vi "r3_HDI&sensor_position_theta.vi"() -> ()   [LabVIEW 2016]
uses:
  Classes/Controllers/Motion/Copy of Motion Folder/Motion.lvclass
  Classes/Controllers/Camera/Copy of Controller Folder/Controller.lvclass
panel:
  in  "Default sensor size type B size":dbl[](array[numeric])=[22.4, 102.0, 78.448, -0.011805]
  in  "Default sensor size type A size":dbl[](array[numeric])=[22.4, 130.0, 78.448, -0.011805]
  in  "Default HDI type A size 2":dbl[](array[numeric])=[24.3, 129.2, 78.448, -0.011805]
  in  "Default HDI type B size":dbl[](array[numeric])=[24.3, 101.2, 78.448, -0.011805]
  in  "Default sensor crossmark \nposition 2":dbl[](array[numeric])=[293.153, 988.113, 78.448, -0.011805]
  in  "Default sensor crossmark \nposition 1":dbl[](array[numeric])=[293.114, 1090.236, 78.428, -0.011805]
  in  "Default HDI alignment \nmark position 2":dbl[](array[numeric])=[292.408, 988.669, 78.824, -0.011805]
  in  "Default HDI alignment \nmark position":dbl[](array[numeric])=[292.414, 1090.827, 78.808, -0.011805]
  out "Type B rotation error":dbl format="%#_8e"
  out "Type B Y error":dbl format="%#_8g"
  out "Type B X error":dbl format="%#_8g"
  out "Type A rotation error":dbl format="%#_8e"
  out "Type A Y error":dbl format="%#_8g"
  out "Type A X error":dbl format="%#_8g"
  out "HDI/sesnor array":bool[](array[boolean])
  out "type a/b array":bool[](array[boolean])
  in  "Type A/ Type B":bool
  in  "HDI / Sensor":bool
  out "the copy array":dbl[](array[numeric]) format="%#_8g"
  out "buttom right C":dbl[](array[numeric]) format="%#_8g"
  out "X position":dbl[](array[numeric]) format="%#_8g"
  out "Yposition":dbl[](array[numeric]) format="%#_8g"
  out "A C center point":dbl[](array[numeric]) format="%#_8g"
  out "loop counting":dbl
  out "rotation":dbl[](array[numeric]) format="%#_8g"
  in  "Stop":bool
  in  "DO measurement":bool=TRUE
  out "buttom left B":dbl[](array[numeric]) format="%#_8g"
  out "upper left A":dbl[](array[numeric]) format="%#_8g"
  out "r-phi":dbl[](array[numeric])
  out "A B center point":dbl[](array[numeric])
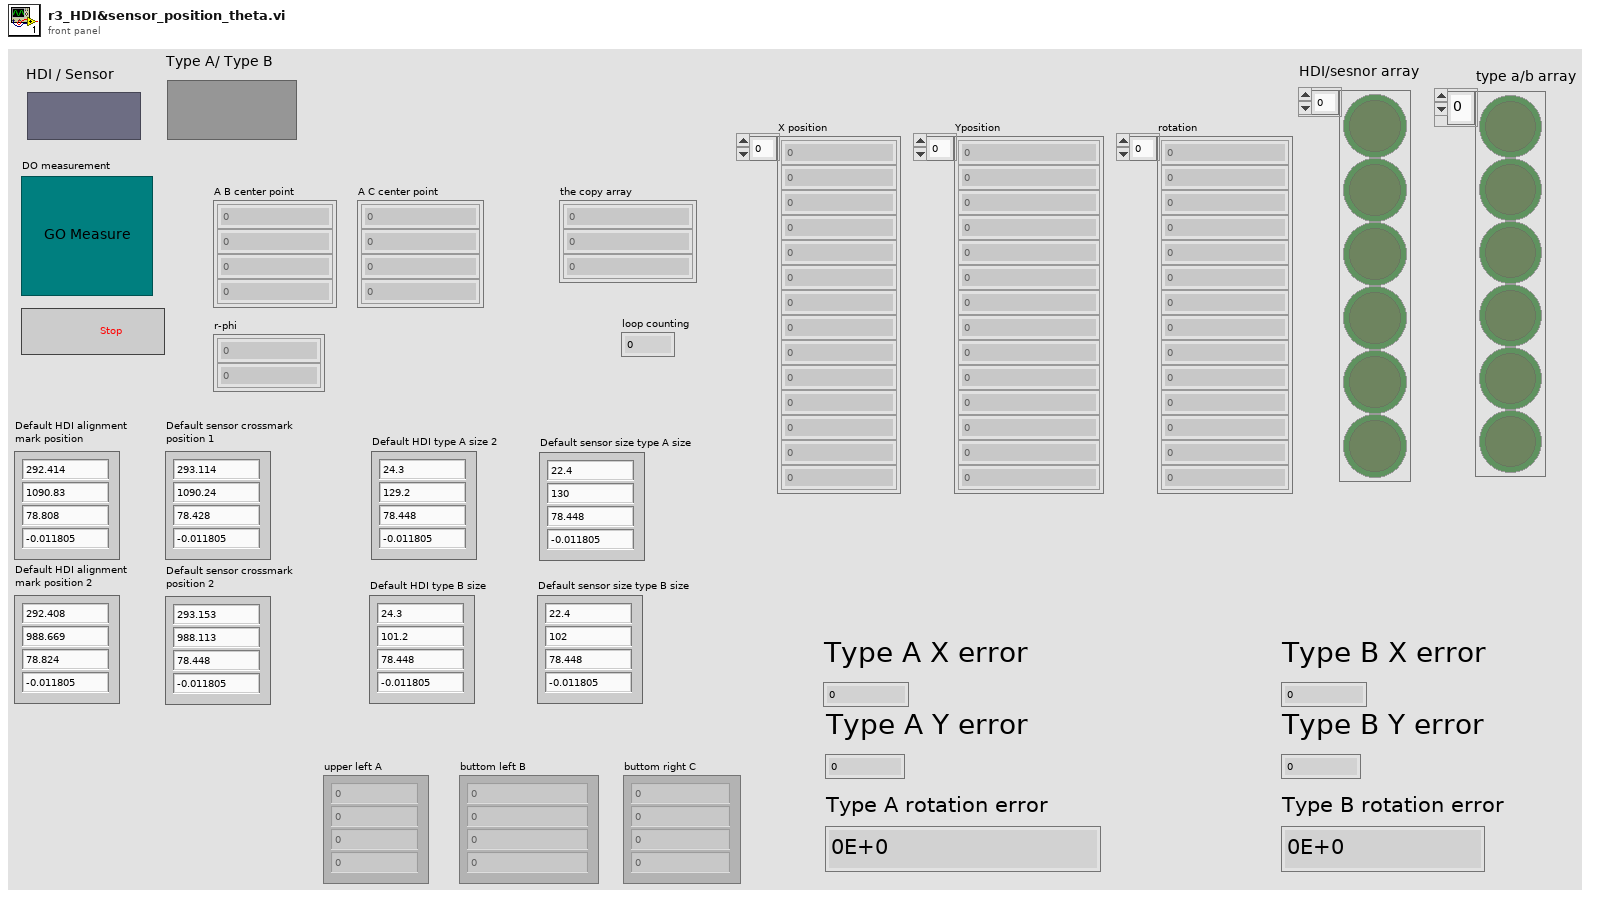
[diagram p1: front panel]
types:
  T1 = typedef "Controller.lvclass/Controllers.ctl" = cluster{"Copy of Motion.lvclass":refnum<class "Motion.lvclass">, "Copy of I-O.lvclass":refnum<class "I-O.lvclass">, "Copy of Dispenser.lvclass":refnum<class "Dispenser.lvclass">}
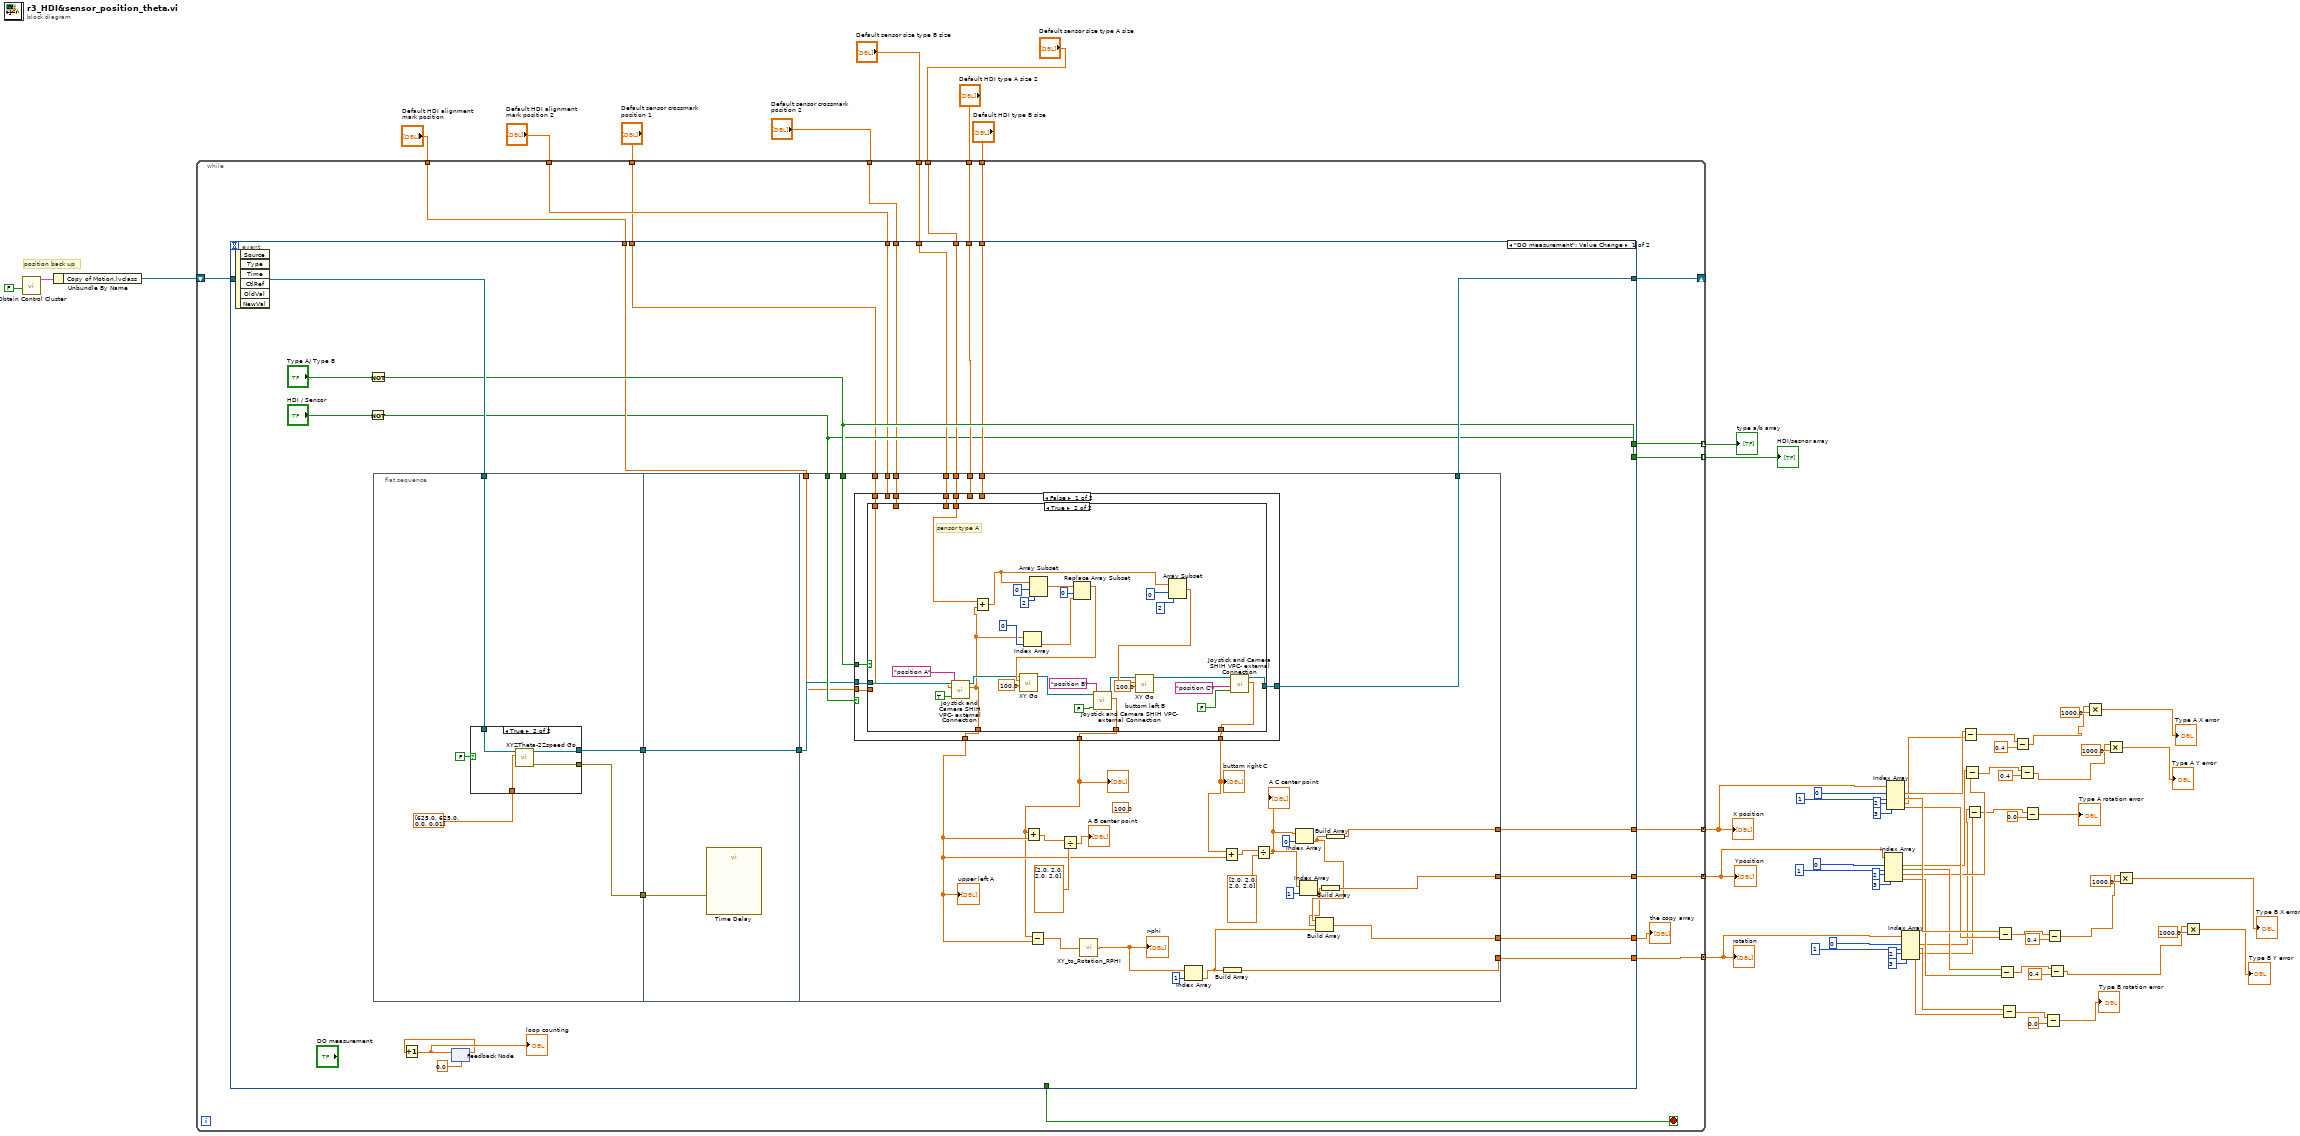
[diagram p0: block diagram]
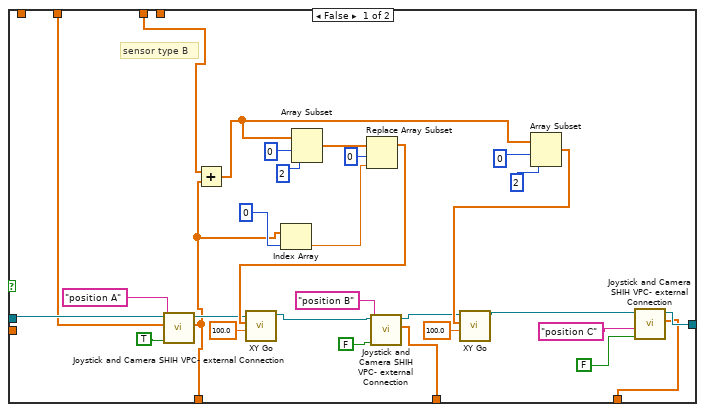
[diagram p3: hidden frame]
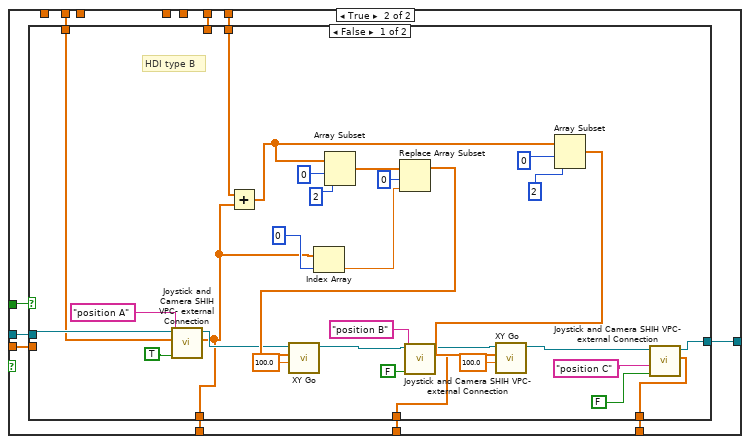
[diagram p4: hidden frame]
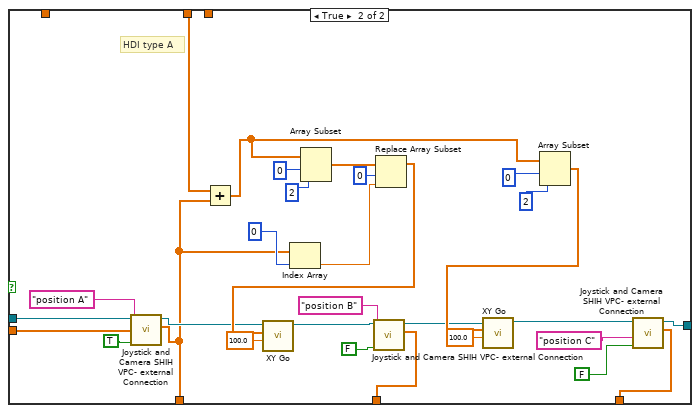
[diagram p5: hidden frame]
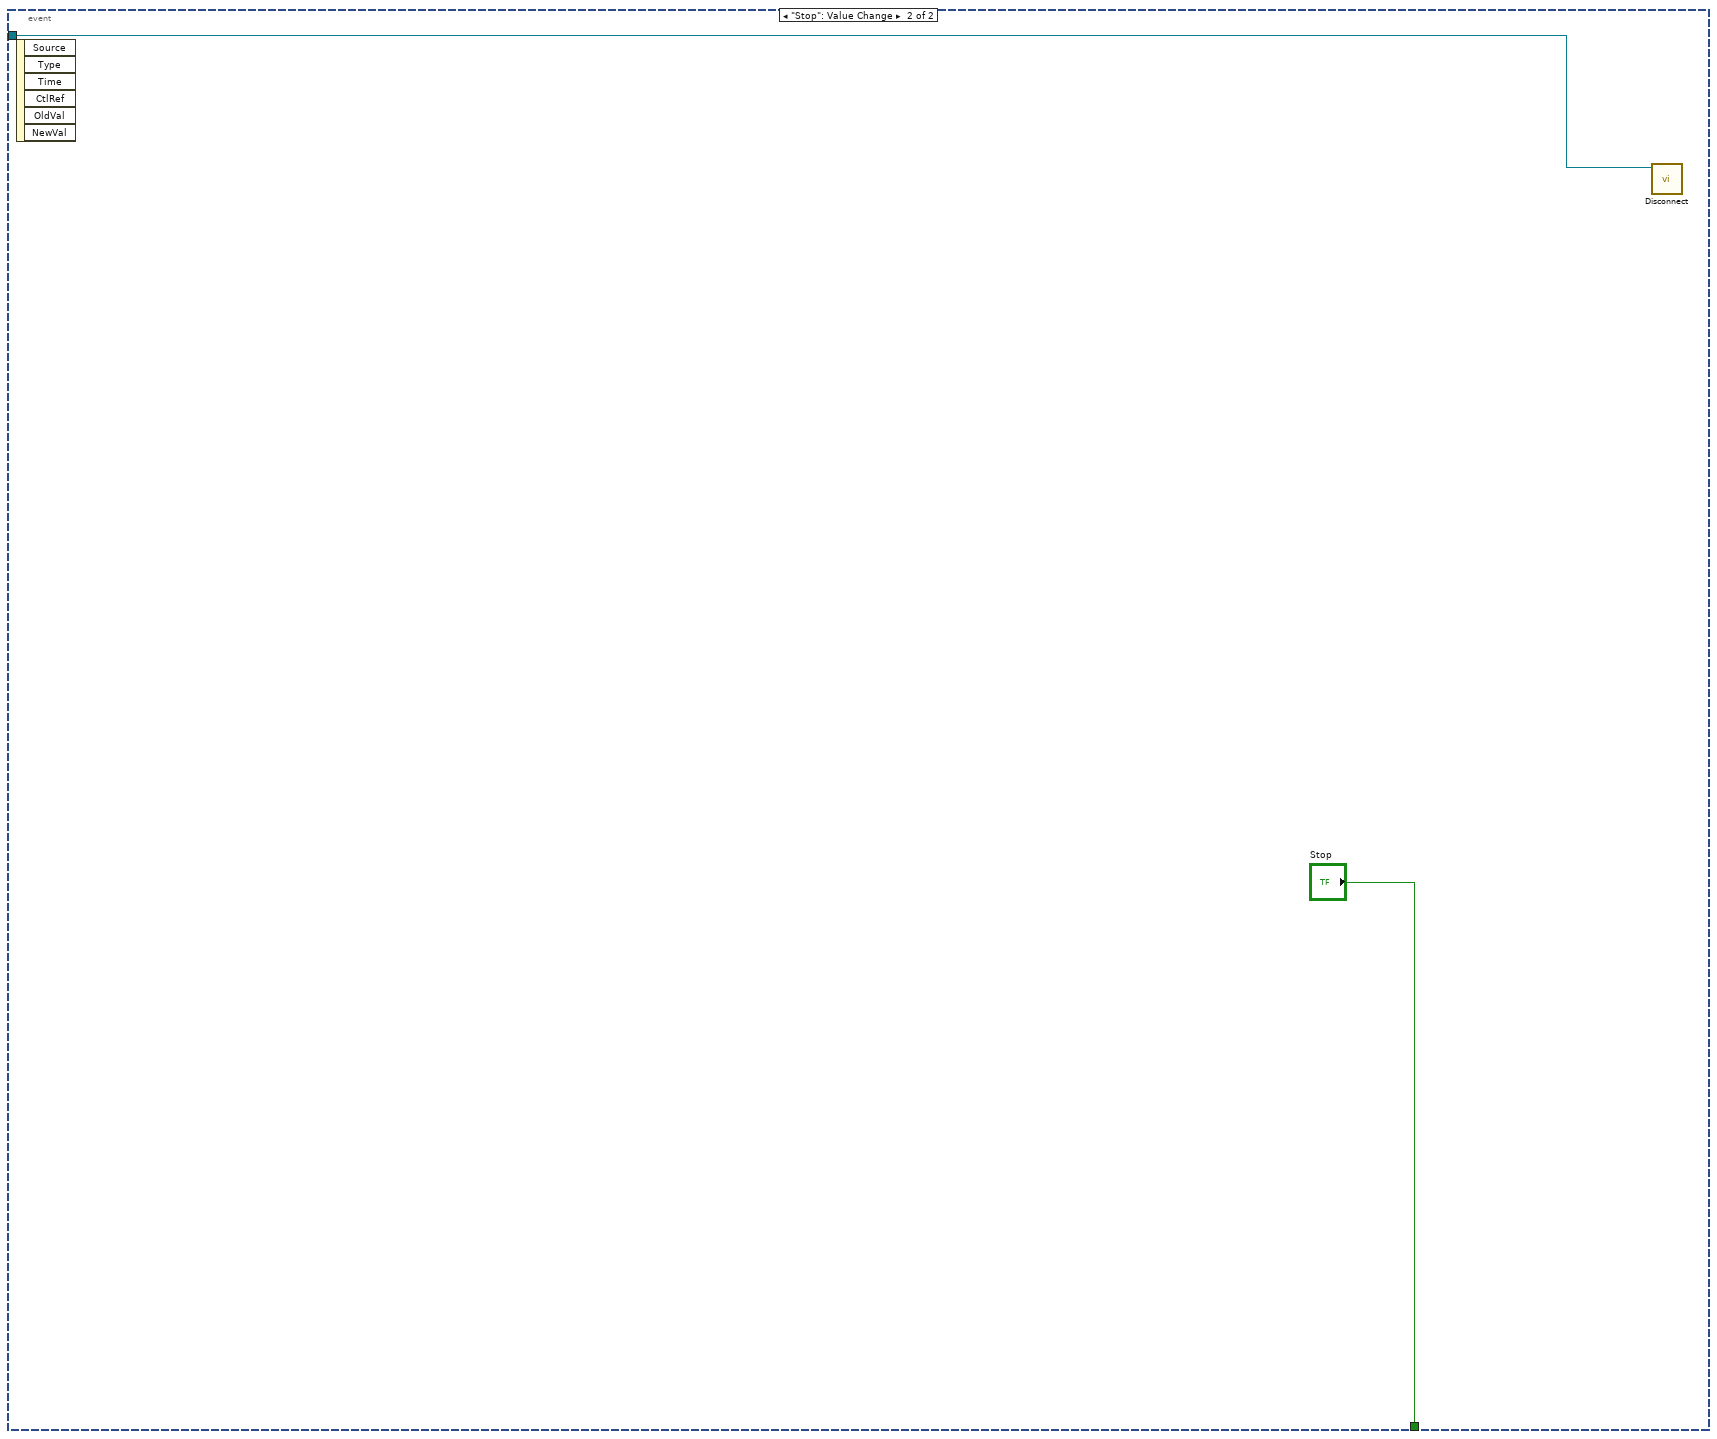
[diagram p6: hidden frame]
diagram:
  # "position back up"
  n1 = call "Obtain Control Cluster.vi"("I/O"=FALSE) -> ("Control Out"=w66:T1)  [unwired: 10 in]
  n2 = Unbundle By Name(w66) -> ("Copy of Motion.lvclass"=w64:refnum<class "Motion.lvclass">)
  n3 = while {
    shift-right: [w81] -> _
    shift-left: w64 -> [w83]
    tunnel: [w80] -> w47 mode=concatenating
    tunnel: [w79] -> w49 mode=concatenating
    tunnel: [w78] -> w48 mode=concatenating
    tunnel: [w76] -> w63 mode=indexing
    tunnel: [w75] -> w62 mode=indexing
    tunnel: "Default HDI type A size 2" -> [w74]
    tunnel: "Default HDI type B size" -> [w73]
    tunnel: "Default sensor size type A size" -> [w72]
    tunnel: "Default sensor size type B size" -> [w71]
    tunnel: "Default HDI alignment \nmark position" -> [w70]
    tunnel: "Default HDI alignment \nmark position 2" -> [w69]
    tunnel: "Default sensor crossmark \nposition 1" -> [w68]
    tunnel: "Default sensor crossmark \nposition 2" -> [w67]
    stop <- w82 stop-if-true
    n4 = event shown="[0] \"DO measurement\": Value Change" {
      selector: _ -> [_ _]
      dyn-events: _ -> [_ _]
      timeout: _ -> [_ _]
      tunnel: w83 -> [w107 w295]
      tunnel: [_ "Stop"] -> w82
      tunnel: [w105 _] -> w81
      tunnel: [w106 _] -> w80
      tunnel: [w101 _] -> w79
      tunnel: [w100 _] -> w78
      tunnel: [w99 _] -> w77
      tunnel: [w96 _] -> w76
      tunnel: [w90 _] -> w75
      tunnel: w74 -> [w95 _]
      tunnel: w73 -> [w94 _]
      tunnel: w72 -> [w93 _]
      tunnel: w71 -> [w92 _]
      tunnel: w70 -> [w91 _]
      tunnel: w69 -> [w86 _]
      tunnel: w68 -> [w85 _]
      tunnel: w67 -> [w84 _]
      event "DO measurement": Value Change {
        n5 = event-data() -> ()  [unwired: 1 in, 6 out]
        n6 = Not(x="HDI / Sensor") -> (.not. x?=w90:bool)
        n7 = Not(x="Type A/ Type B") -> (.not. x?=w96:bool)
        n8 = flat-sequence {
          tunnel: w107 -> [w111]
          tunnel: [w110] -> w89
          tunnel: [w109] -> w88
          tunnel: w89 -> [w119]
          tunnel: [w118] -> w87
          tunnel: w88 -> [w118]
          tunnel: w87 -> [w126]
          tunnel: [w146] -> w106
          tunnel: [w124] -> w105
          tunnel: [w140] -> w101
          tunnel: [w139] -> w100
          tunnel: [w135] -> w99
          tunnel: w90 -> [w134]
          tunnel: w96 -> [w133]
          tunnel: w95 -> [w132]
          tunnel: w94 -> [w131]
          tunnel: w93 -> [w129]
          tunnel: w92 -> [w128]
          tunnel: w91 -> [w125]
          tunnel: w86 -> [w122]
          tunnel: w85 -> [w121]
          tunnel: w84 -> [w120]
          frame #0 {
            n9 = case shown="True" FALSE {
              tunnel: dbl[] [625.0, 625.0, 0.0, 0.01] ("Parking position") -> [_ w117]
              tunnel: w111 -> [w113 w116]
              tunnel: [_ w115] -> w110
              tunnel: [w113 w114] -> w109
              frame False {
              }
              frame True {
                n10 = call "XYZTheta-2Zspeed Go.vi"("XYZTheta In"=w117, "Motion in"=w116) -> ("error out"=w115:errorcluster, "Motion out"=w114:refnum<class "Motion.lvclass">)  [unwired: 7 in, 1 out]
              }
            }
          }
          frame #1 {
            n11 = call "Time Delay"("error in (no error)"=w119) -> ()  [unwired: 10 in, 1 out]
          }
          frame #2 {
            (unwired) 100.0 ("Speed")
            n12 = case shown="False" w134 {
              tunnel: w133 -> [w163 w233]
              tunnel: w132 -> [_ w232]
              tunnel: w131 -> [_ w231]
              tunnel: [w158 w230] -> w130
              tunnel: w129 -> [w162 _]
              tunnel: w128 -> [w161 _]
              tunnel: [w157 w229] -> w127
              tunnel: w126 -> [w160 w228]
              tunnel: w125 -> [w159 w227]
              tunnel: [w155 w226] -> w124
              tunnel: [w156 w225] -> w123
              tunnel: w122 -> [_ w224]
              tunnel: w121 -> [w154 _]
              tunnel: w120 -> [w153 _]
              frame False {
                n13 = case shown="True" w163 {
                  tunnel: w162 -> [_ w215]
                  tunnel: w161 -> [w185 _]
                  tunnel: w160 -> [w178 w208]
                  tunnel: w159 -> [_ _]
                  tunnel: [w166 w196] -> w158
                  tunnel: [w173 w202] -> w157
                  tunnel: [w167 w198] -> w156
                  tunnel: [w168 w197] -> w155
                  tunnel: w154 -> [_ w194]
                  tunnel: w153 -> [w164 _]
                  frame False {
                    # "sensor type B"
                    n14 = call "Joystick and Camera SHIH VPC- external Connection.vi"("Motion in"=w178, "XYZTheta"=w164, "Measurement Point"="position A", "Inital GO"=TRUE) -> ("Motion out"=w177:refnum<class "Motion.lvclass">, "Sum"=w166:dbl[])  [unwired: 3 in, 2 out]
                    n15 = Add(x=w185, y=w166) -> (x+y=w190:dbl[])
                    n16 = Index Array(array=w166, index=0) -> (element=w165:dbl)
                    n17 = Array Subset(array=w190, index=0, length=2) -> (w191:dbl[])
                    n18 = Replace Array Subset(array=w191, new element=w165, index=0) -> (w184:dbl[])
                    n19 = call-dynamic "XY Go.vi"("Speed"=100.0, "XY"=w184, "Motion in"=w177) -> ("Motion out"=w174:refnum<class "Motion.lvclass">)  [unwired: 7 in, 1 out]
                    n20 = call "Joystick and Camera SHIH VPC- external Connection.vi"("Motion in"=w174, "Measurement Point"="position B", "Inital GO"=FALSE) -> ("Motion out"=w172:refnum<class "Motion.lvclass">, "Sum"=w173:dbl[])  [unwired: 4 in, 2 out]
                    n21 = Array Subset(array=w190, index=0, length=2) -> (w183:dbl[])
                    n22 = call-dynamic "XY Go.vi"("Speed"=100.0, "XY"=w183, "Motion in"=w172) -> ("Motion out"=w169:refnum<class "Motion.lvclass">)  [unwired: 7 in, 1 out]
                    n23 = call "Joystick and Camera SHIH VPC- external Connection.vi"("Motion in"=w169, "Measurement Point"="position C", "Inital GO"=FALSE) -> ("Motion out"=w168:refnum<class "Motion.lvclass">, "Sum"=w167:dbl[])  [unwired: 4 in, 2 out]
                  }
                  frame True {
                    # "sensor type A"
                    n24 = call "Joystick and Camera SHIH VPC- external Connection.vi"("Motion in"=w208, "XYZTheta"=w194, "Measurement Point"="position A", "Inital GO"=TRUE) -> ("Motion out"=w207:refnum<class "Motion.lvclass">, "Sum"=w196:dbl[])  [unwired: 3 in, 2 out]
                    n25 = Add(x=w215, y=w196) -> (x+y=w219:dbl[])
                    n26 = Index Array(array=w196, index=0) -> (element=w195:dbl)
                    n27 = Array Subset(array=w219, index=0, length=2) -> (w218:dbl[])
                    n28 = Replace Array Subset(array=w218, new element=w195, index=0) -> (w214:dbl[])
                    n29 = call-dynamic "XY Go.vi"("Speed"=100.0, "XY"=w214, "Motion in"=w207) -> ("Motion out"=w204:refnum<class "Motion.lvclass">)  [unwired: 7 in, 1 out]
                    n30 = call "Joystick and Camera SHIH VPC- external Connection.vi"("Motion in"=w204, "Measurement Point"="position B", "Inital GO"=FALSE) -> ("Motion out"=w203:refnum<class "Motion.lvclass">, "Sum"=w202:dbl[])  [unwired: 4 in, 2 out]
                    n31 = Array Subset(array=w219, index=0, length=2) -> (w213:dbl[])
                    n32 = call-dynamic "XY Go.vi"("Speed"=100.0, "XY"=w213, "Motion in"=w203) -> ("Motion out"=w199:refnum<class "Motion.lvclass">)  [unwired: 7 in, 1 out]
                    n33 = call "Joystick and Camera SHIH VPC- external Connection.vi"("Motion in"=w199, "Measurement Point"="position C", "Inital GO"=FALSE) -> ("Motion out"=w197:refnum<class "Motion.lvclass">, "Sum"=w198:dbl[])  [unwired: 4 in, 2 out]
                  }
                }
              }
              frame True {
                n34 = case shown="False" w233 {
                  tunnel: w232 -> [_ w285]
                  tunnel: w231 -> [w255 _]
                  tunnel: [w236 w270] -> w230
                  tunnel: [w243 w278] -> w229
                  tunnel: w228 -> [w247 w273]
                  tunnel: w227 -> [_ w272]
                  tunnel: [w238 w266] -> w226
                  tunnel: [w237 w264] -> w225
                  tunnel: w224 -> [w234 _]
                  frame False {
                    # "HDI type B"
                    n35 = call "Joystick and Camera SHIH VPC- external Connection.vi"("Motion in"=w247, "XYZTheta"=w234, "Measurement Point"="position A", "Inital GO"=TRUE) -> ("Motion out"=w248:refnum<class "Motion.lvclass">, "Sum"=w236:dbl[])  [unwired: 3 in, 2 out]
                    n36 = Add(x=w255, y=w236) -> (x+y=w259:dbl[])
                    n37 = Index Array(array=w236, index=0) -> (element=w235:dbl)
                    n38 = Array Subset(array=w259, index=0, length=2) -> (w258:dbl[])
                    n39 = Replace Array Subset(array=w258, new element=w235, index=0) -> (w254:dbl[])
                    n40 = call-dynamic "XY Go.vi"("Speed"=100.0, "XY"=w254, "Motion in"=w248) -> ("Motion out"=w245:refnum<class "Motion.lvclass">)  [unwired: 7 in, 1 out]
                    n41 = call "Joystick and Camera SHIH VPC- external Connection.vi"("Motion in"=w245, "Measurement Point"="position B", "Inital GO"=FALSE) -> ("Motion out"=w244:refnum<class "Motion.lvclass">, "Sum"=w243:dbl[])  [unwired: 4 in, 2 out]
                    n42 = Array Subset(array=w259, index=0, length=2) -> (w253:dbl[])
                    n43 = call-dynamic "XY Go.vi"("Speed"=100.0, "XY"=w253, "Motion in"=w244) -> ("Motion out"=w239:refnum<class "Motion.lvclass">)  [unwired: 7 in, 1 out]
                    n44 = call "Joystick and Camera SHIH VPC- external Connection.vi"("Motion in"=w239, "Measurement Point"="position C", "Inital GO"=FALSE) -> ("Motion out"=w238:refnum<class "Motion.lvclass">, "Sum"=w237:dbl[])  [unwired: 4 in, 2 out]
                  }
                  frame True {
                    # "HDI type A"
                    n45 = call "Joystick and Camera SHIH VPC- external Connection.vi"("Motion in"=w273, "XYZTheta"=w272, "Measurement Point"="position A", "Inital GO"=TRUE) -> ("Motion out"=w271:refnum<class "Motion.lvclass">, "Sum"=w270:dbl[])  [unwired: 3 in, 2 out]
                    n46 = Add(x=w285, y=w270) -> (x+y=w289:dbl[])
                    n47 = Index Array(array=w270, index=0) -> (element=w284:dbl)
                    n48 = Array Subset(array=w289, index=0, length=2) -> (w288:dbl[])
                    n49 = Replace Array Subset(array=w288, new element=w284, index=0) -> (w283:dbl[])
                    n50 = call-dynamic "XY Go.vi"("Speed"=100.0, "XY"=w283, "Motion in"=w271) -> ("Motion out"=w277:refnum<class "Motion.lvclass">)  [unwired: 7 in, 1 out]
                    n51 = call "Joystick and Camera SHIH VPC- external Connection.vi"("Motion in"=w277, "Measurement Point"="position B", "Inital GO"=FALSE) -> ("Motion out"=w276:refnum<class "Motion.lvclass">, "Sum"=w278:dbl[])  [unwired: 4 in, 2 out]
                    n52 = Array Subset(array=w289, index=0, length=2) -> (w282:dbl[])
                    n53 = call-dynamic "XY Go.vi"("Speed"=100.0, "XY"=w282, "Motion in"=w276) -> ("Motion out"=w267:refnum<class "Motion.lvclass">)  [unwired: 7 in, 1 out]
                    n54 = call "Joystick and Camera SHIH VPC- external Connection.vi"("Motion in"=w267, "Measurement Point"="position C", "Inital GO"=FALSE) -> ("Motion out"=w266:refnum<class "Motion.lvclass">, "Sum"=w264:dbl[])  [unwired: 4 in, 2 out]
                  }
                }
              }
            }
            "upper left A" <- w130
            "buttom left B" <- w127
            "buttom right C" <- w123
            n55 = Add(x=w127, y=w130) -> (x+y=w149:dbl[])
            n56 = Subtract(x=w127, y=w130) -> (x-y=w152:dbl[])
            n57 = Divide(x=w149, y=dbl[] [2.0, 2.0, 2.0, 2.0]) -> (x/y=→"A B center point":dbl[])
            n58 = call "XY_to_Rotation_RPHI.vi"("X-Y"=w152) -> ("r-phi"=w147:dbl[])
            "r-phi" <- w147
            n59 = Index Array(array=w147, index=1) -> (element=w136:dbl)
            n60 = Add(x=w123, y=w130) -> (x+y=w144:dbl[])
            n61 = Build Array(w136) -> (w146:dbl[])
            n62 = Divide(x=w144, y=dbl[] [2.0, 2.0, 2.0, 2.0]) -> (x/y=w141:dbl[])
            "A C center point" <- w141
            n63 = Index Array(array=w141, index=0) -> (element=w138:dbl)
            n64 = Index Array(array=w141, index=1) -> (element=w137:dbl)
            n65 = Build Array(w138, w137, w136) -> (w135:dbl[])
            n66 = Build Array(w137) -> (w139:dbl[])
            n67 = Build Array(w138) -> (w140:dbl[])
          }
        }
        n68 = feedback #1(0.0) -> (w102:dbl)
        n69 = Increment(x=w102) -> (x+1=w104:dbl)
        "loop counting" <- w104
        n70 = feedback-in #1(w104) -> ()
      }
      event "Stop": Value Change {
        n71 = event-data() -> ()  [unwired: 1 in, 6 out]
        n72 = call-dynamic "Disconnect.vi"("Controller in"=w295) -> ()  [unwired: 9 in, 1 out]
      }
    }
    "the copy array" <- w77
  }
  "rotation" <- w47
  "X position" <- w49
  "Yposition" <- w48
  "type a/b array" <- w63
  "HDI/sesnor array" <- w62
  n73 = Index Array(array=w48, index #1=0 ("index"), index #2=1 ("index"), index #3=2 ("index"), index #4=3 ("index")) -> (element #1=w42:dbl, element #2=w41:dbl, element #3=w40:dbl, element #4=w39:dbl)
  n74 = Index Array(array=w49, index #1=0 ("index"), index #2=1 ("index"), index #3=2 ("index"), index #4=3 ("index")) -> (element #1=w46:dbl, element #2=w45:dbl, element #3=w44:dbl, element #4=w43:dbl)
  n75 = Index Array(array=w47, index #1=0 ("index"), index #2=1 ("index"), index #3=2 ("index"), index #4=3 ("index")) -> (element #1=w38:dbl, element #2=w37:dbl, element #3=w36:dbl, element #4=w35:dbl)
  n76 = Subtract(x=w46, y=w44) -> (x-y=w28:dbl)
  n77 = Subtract(x=w42, y=w40) -> (x-y=w27:dbl)
  n78 = Subtract(x=w38, y=w36) -> (x-y=w26:dbl)
  n79 = Subtract(x=w45, y=w43) -> (x-y=w25:dbl)
  n80 = Subtract(x=w41, y=w39) -> (x-y=w24:dbl)
  n81 = Subtract(x=w37, y=w35) -> (x-y=w23:dbl)
  n82 = Subtract(x=w28, y=0.4) -> (x-y=w19:dbl)
  n83 = Subtract(x=w27, y=0.4) -> (x-y=w16:dbl)
  n84 = Subtract(x=w26, y=0.0) -> (x-y=→"Type A rotation error":dbl)
  n85 = Subtract(x=w23, y=0.0) -> (x-y=→"Type B rotation error":dbl)
  n86 = Subtract(x=w25, y=0.4) -> (x-y=w13:dbl)
  n87 = Subtract(x=w24, y=0.4) -> (x-y=w10:dbl)
  n88 = Multiply(x=w19, y=1000.0) -> (x*y=→"Type A X error":dbl)
  n89 = Multiply(x=w16, y=1000.0) -> (x*y=→"Type A Y error":dbl)
  n90 = Multiply(x=w13, y=1000.0) -> (x*y=→"Type B X error":dbl)
  n91 = Multiply(x=w10, y=1000.0) -> (x*y=→"Type B Y error":dbl)
